vi "Inst_DS360.vi"(8 "error in":errorcluster, 10 "All Message Queues in":T1, 11 "Prueba31 in":refnum<class "Prueba03.lvclass">) -> (0 "error out":errorcluster)   [LabVIEW 2019, in "Prueba03.lvclass"]
uses:
  Prueba03.lvclass
  QMH/Message Queue/All Message Queues.ctl
  QMH/Message Queue/Message Cluster.ctl
  Prueba03.lvclass/Prueba03.ctl
  <vilib>/Utility/error.llb/Error Cluster From Error Code.vi
  QMH/Message Queue/Enqueue Message (Single).vi
  <vilib>/ErrorRing/Error Ring.xnode
  QMH/Message Queue/Message Queue.lvlib
  Instrumento/DS360/DS360.lvclass
panel:
  out "All States":string[](array[string])
  out "Actual State":string
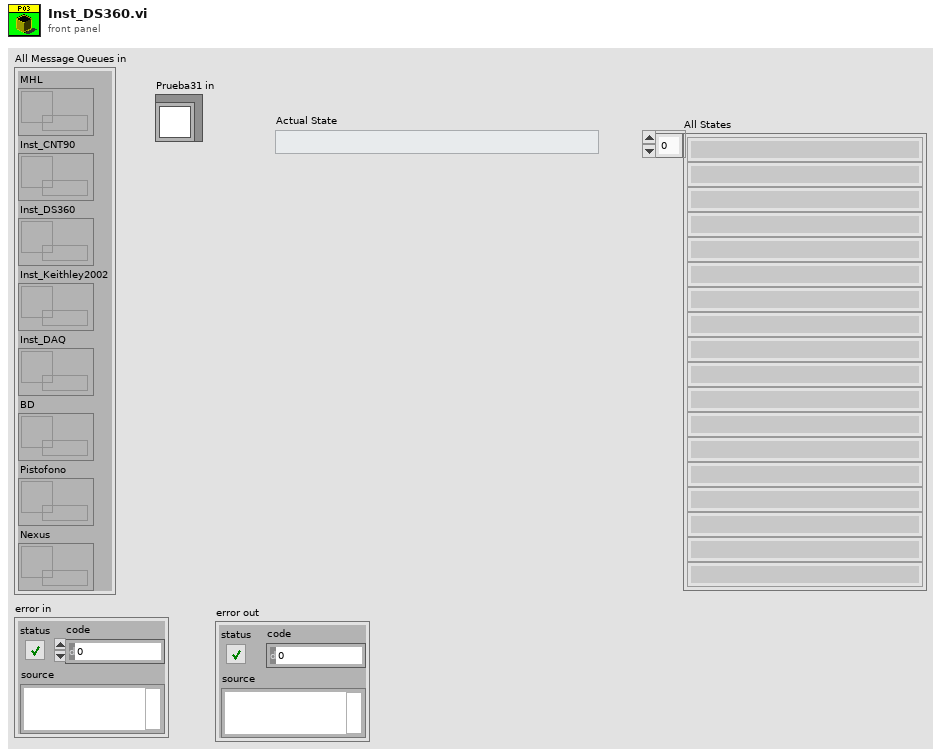
[diagram p1: front panel]
types:
  T1 = typedef "Message Queue.lvlib/All Message Queues.ctl" = cluster{"MHL":refnum<queue>, "Inst_CNT90":refnum<queue>, "Inst_DS360":refnum<queue>, "Inst_Keithley2002":refnum<queue>, "Inst_DAQ":refnum<queue>, "BD":refnum<queue>, "Pistofono":refnum<queue>, "Nexus":refnum<queue>}
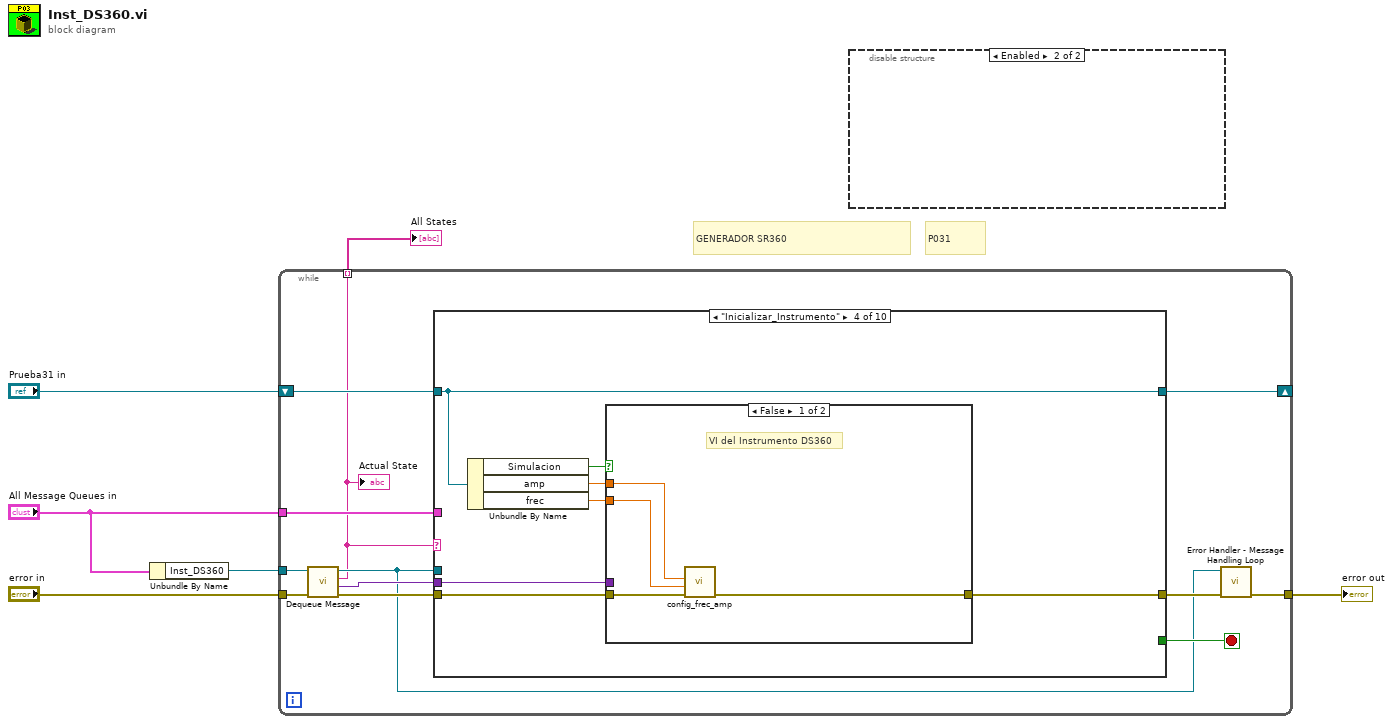
[diagram p0: block diagram]
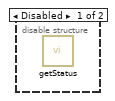
[diagram p2: hidden frame]
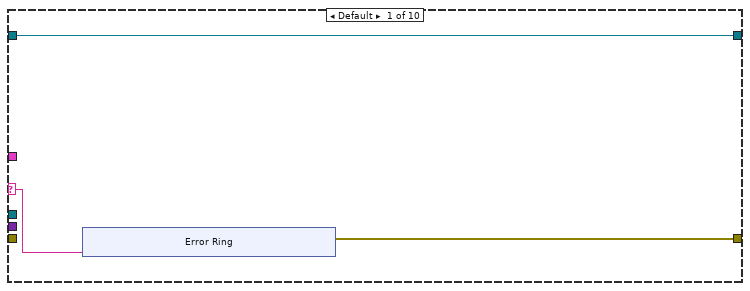
[diagram p3: hidden frame]
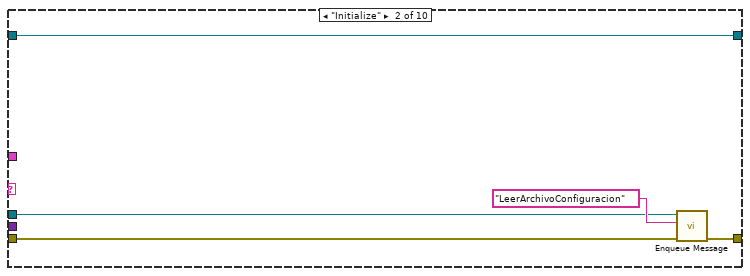
[diagram p4: hidden frame]
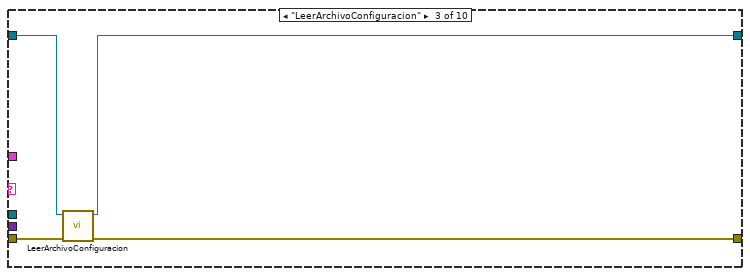
[diagram p5: hidden frame]
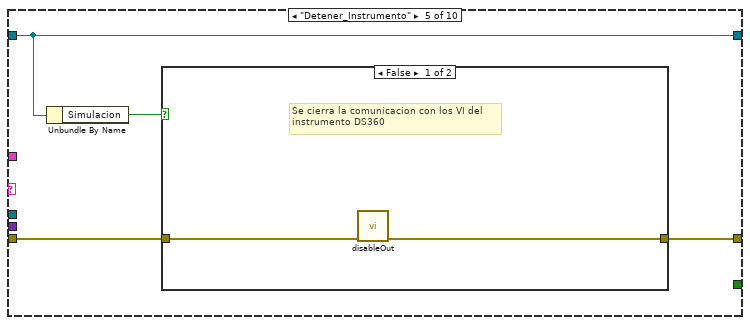
[diagram p7: hidden frame]
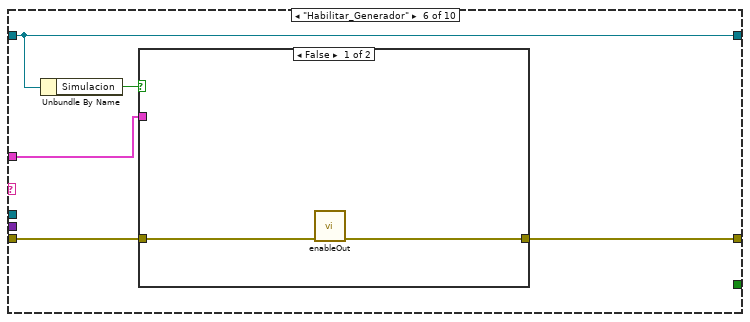
[diagram p9: hidden frame]
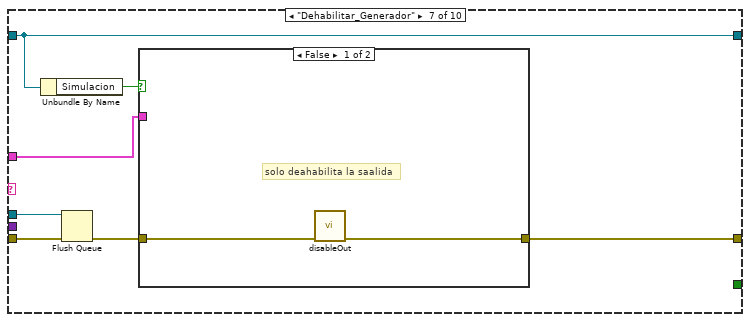
[diagram p11: hidden frame]
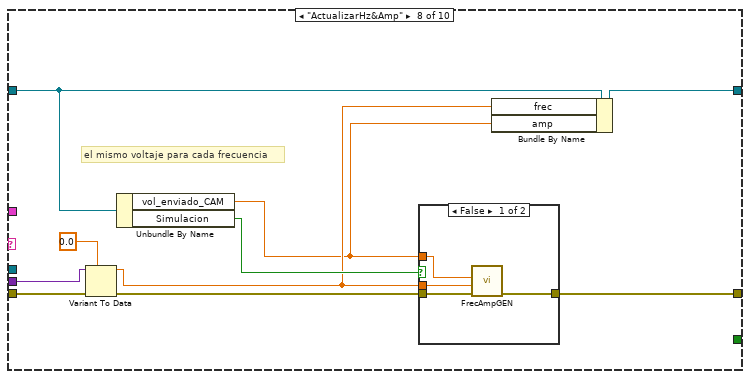
[diagram p13: hidden frame]
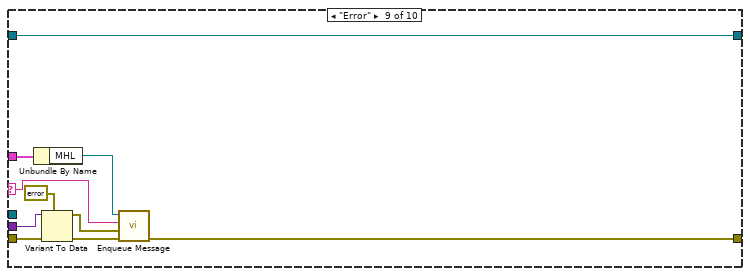
[diagram p15: hidden frame]
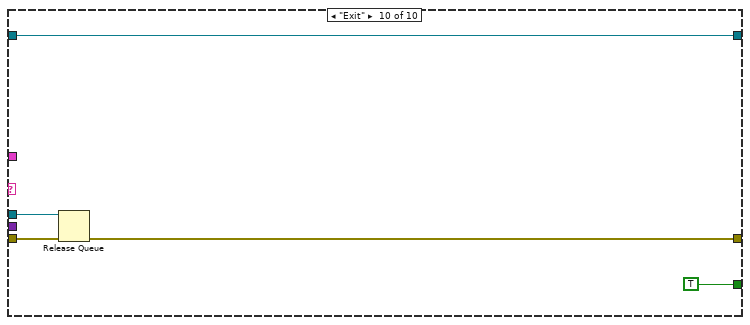
[diagram p16: hidden frame]
diagram:
  # "P031"
  # "GENERADOR SR360"
  n1 = Unbundle By Name("All Message Queues in") -> ("Inst_DS360"=w4:refnum<queue>)
  n2 = while {
    tunnel: "error in" -> [w18]
    tunnel: w4 -> [w17]
    tunnel: "All Message Queues in" -> [w16]
    tunnel: [w9] -> w2
    shift-right: [w12] -> _
    shift-left: "Prueba31 in" -> [w15]
    tunnel: [w7] -> w1 mode=indexing
    stop <- w11 stop-if-true
    n3 = call "Dequeue Message.vi"("error in (no error)"=w18, "Message Queue"=w17) -> ("error out"=w13:errorcluster, "Message Data"=w14:variant, "Message"=w7:string, "dup Message Queue"=w8:refnum<queue>)  [unwired: 6 in]
    "Actual State" <- w7
    n4 = case shown="\"Inicializar_Instrumento\"" w7 {
      selector: w7 -> [w21 _ _ _ _ _ _ _ w92 _]
      tunnel: w16 -> [_ _ _ _ _ w60 w70 _ w91 _]
      tunnel: w15 -> [w19 w33 w34 w42 w52 w59 w69 w80 w99 w101]
      tunnel: w8 -> [_ w29 _ _ _ _ w65 _ _ w103]
      tunnel: w14 -> [_ _ _ w41 _ _ _ w81 w96 _]
      tunnel: w13 -> [_ w30 w36 w40 w50 w61 w71 w82 w97 w104]
      tunnel: [w20 w31 w37 w44 w53 w57 w67 w84 w94 w100] -> w10
      tunnel: [w19 w33 w35 w42 w52 w59 w69 w77 w99 w101] -> w12
      tunnel: [_ _ _ _ _ _ _ _ _ TRUE] -> w11
      frame Default {
        n5 = xnode "Error Ring"("parameter 0"=w21) -> ("error out"=w20:errorcluster)
      }
      frame "Initialize" {
        n6 = call-poly "Enqueue Message.vi"("error in (no error)"=w30, "Message"="LeerArchivoConfiguracion", "Message Queue"=w29) -> ("error out"=w31:errorcluster)  [unwired: 7 in, 1 out]
      }
      frame "LeerArchivoConfiguracion" {
        n7 = call "LeerArchivoConfiguracion.vi"("error in"=w36, "Prueba31 in"=w34) -> ("error out"=w37:errorcluster, "Prueba31 out"=w35:refnum<class "Prueba03.lvclass">)  [unwired: 8 in]
      }
      frame "Inicializar_Instrumento" {
        n8 = Unbundle By Name(w42) -> ("Simulacion"=w43:bool, "amp"=w39:dbl, "frec"=w38:dbl)
        n9 = case shown="False" w43 {
          tunnel: [w47 w49] -> w44
          tunnel: w40 -> [w48 w49]
          tunnel: w41 -> [_ _]
          tunnel: w39 -> [w46 _]
          tunnel: w38 -> [w45 _]
          frame False {
            # "VI del Instrumento DS360"
            n10 = call "config_frec_amp.vi"("error in (no error)"=w48, "Frec (Hz)"=w45, "Amplitud (Vrms)"=w46) -> ("error out"=w47:errorcluster)  [unwired: 7 in, 1 out]
          }
          frame True {
            # "Simulacion"
          }
        }
      }
      frame "Detener_Instrumento" {
        n11 = Unbundle By Name(w52) -> ("Simulacion"=w51:bool)
        n12 = case shown="False" w51 {
          tunnel: [w55 w56] -> w53
          tunnel: w50 -> [w54 w56]
          frame False {
            # "Se cierra la comunicacion con los VI del\ninstrumento DS360"
            n13 = call "disableOut.vi"("error in (no error)"=w54) -> ("error out"=w55:errorcluster)  [unwired: 9 in, 1 out]
          }
          frame True {
            # "Simulacion"
          }
        }
      }
      frame "Habilitar_Generador" {
        n14 = Unbundle By Name(w59) -> ("Simulacion"=w58:bool)
        n15 = case shown="False" w58 {
          tunnel: [w62 w64] -> w57
          tunnel: w61 -> [w63 w64]
          tunnel: w60 -> [_ _]
          frame False {
            n16 = call "enableOut.vi"("error in (no error)"=w63) -> ("error out"=w62:errorcluster)  [unwired: 9 in, 1 out]
          }
          frame True {
          }
        }
      }
      frame "Dehabilitar_Generador" {
        n17 = Unbundle By Name(w69) -> ("Simulacion"=w68:bool)
        n18 = Flush Queue(queue=w65, error in (no error)=w71) -> (error out=w66:errorcluster)  [unwired: 2 out]
        n19 = case shown="False" w68 {
          tunnel: [w72 w74] -> w67
          tunnel: w66 -> [w73 w74]
          tunnel: w70 -> [_ _]
          frame False {
            # "solo deahabilita la saalida"
            n20 = call "disableOut.vi"("error in (no error)"=w73) -> ("error out"=w72:errorcluster)  [unwired: 9 in, 1 out]
          }
          frame True {
          }
        }
      }
      frame "ActualizarHz&Amp" {
        # "el mismo voltaje para cada frecuencia"
        n21 = Variant To Data(error in=w82, type=0.0, Variant=w81) -> (data=w76:dbl, error out=w83:errorcluster)
        n22 = Unbundle By Name(w80) -> ("vol_enviado_CAM"=w75:dbl, "Simulacion"=w78:bool)
        n23 = case shown="False" w78 {
          tunnel: [w88 w89] -> w84
          tunnel: w83 -> [w87 w89]
          tunnel: w75 -> [w86 _]
          tunnel: w76 -> [w85 _]
          frame False {
            n24 = call "FrecAmpGEN.vi"("error in (no error)"=w87, "Frec (Hz)"=w85, "Amplitud (Vrms)"=w86) -> ("error out"=w88:errorcluster)  [unwired: 7 in, 1 out]
          }
          frame True {
            # "Simlacion"
          }
        }
        n25 = Bundle By Name(cluster=w80, "frec"=w76, "amp"=w75) -> (w77:refnum<class "Prueba03.lvclass">)
      }
      frame "Error" {
        n26 = Unbundle By Name(w91) -> ("MHL"=w90:refnum<queue>)
        n27 = Variant To Data(error in=w97, type=errorcluster {"status"=FALSE, "code"=0, "source"=""} ("error constant"), Variant=w96) -> (data=w93:errorcluster, error out=w95:errorcluster)
        n28 = call-poly "Enqueue Message.vi"("error in (no error)"=w95, "Message Data"=w93, "Message"=w92, "Message Queue"=w90) -> ("error out"=w94:errorcluster)  [unwired: 6 in, 1 out]
      }
      frame "Exit" {
        n29 = Release Queue(queue=w103, error in (no error)=w104) -> (error out=w100:errorcluster)  [unwired: 1 in, 2 out]
      }
    }
    n30 = call "Error Handler - Message Handling Loop.vi"("error in (no error)"=w10, "Message Queue"=w8) -> ("dup error in"=w9:errorcluster)  [unwired: 8 in, 1 out]
  }
  "error out" <- w2
  "All States" <- w1
  n31 = disable-structure shown="Enabled" {
    frame Disabled {
      n32 = call "getStatus.vi"() -> ()  [unwired: 9 in, 3 out]
    }
    frame Enabled {
    }
  }
